vi "Inform.vi"(8 "error in (no error)":errorcluster, 10 "Message in":refnum<class "InformMessage.lvclass">, 11 "ServiceManager in":refnum<class "ServiceManager.lvclass">) -> (0 "error out":errorcluster, 3 "ServiceManager out":refnum<class "ServiceManager.lvclass">)   [LabVIEW 2012, in "ServiceManager.lvclass"]
doc: "The inform method processes the command inform'. \n\nThe command inform' is used for obtaining the latest instance data of the class. It also handles the current state of the observee and sets the 'ready' flag for the observee."
uses:
  ServiceManager.lvclass
  Murmex/LabVIEW/Murmex/InformMessage/InformMessage.lvclass
  Murmex/LabVIEW/Murmex/Murmex/Murmex.lvclass
  Murmex/LabVIEW/Murmex/Murmex/status_enum.ctl
  ServiceManager.lvclass/ServiceManager.ctl
  boot_parameters_cluster.ctl
  Murmex/LabVIEW/Murmex/Murmex/component_specification_cluster.ctl
  Murmex/LabVIEW/Murmex/GenericMessage/GenericMessage.lvclass
  Murmex/LabVIEW/Murmex/Message/Message.lvclass
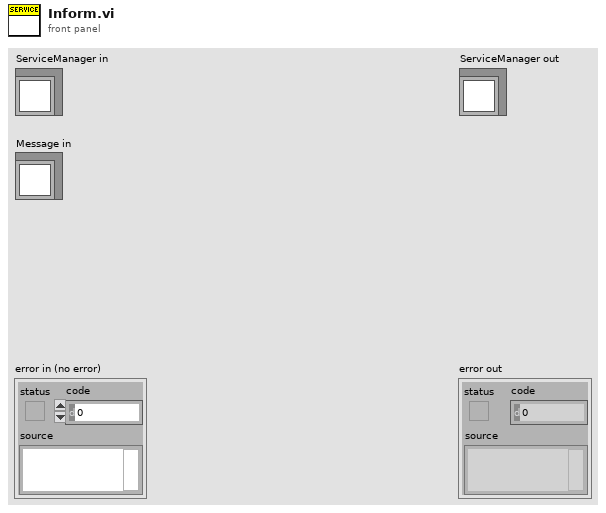
[diagram p1: front panel]
types:
  T1 = typedef "Murmex.lvlib/Murmex.lvclass/status_enum.ctl" = enum16{"ready", "warning", "error", "shutting down", "initialising"}
  T2 = typedef "ServiceManager.lvclass/boot_parameters_cluster.ctl" = cluster{"component specification":T3, "search paths":cluster{"path":string[]}}
  T3 = typedef "Murmex.lvlib/Murmex.lvclass/component_specification_cluster.ctl" = cluster{"name":string, "language":string, "host name":string, "id":string}
  T4 = typedef "ServiceManager.lvclass/loaded_components_cluster.ctl" = cluster{"component specification":T3, "booted?":bool, "status":T1, "last seen?":timestamp}
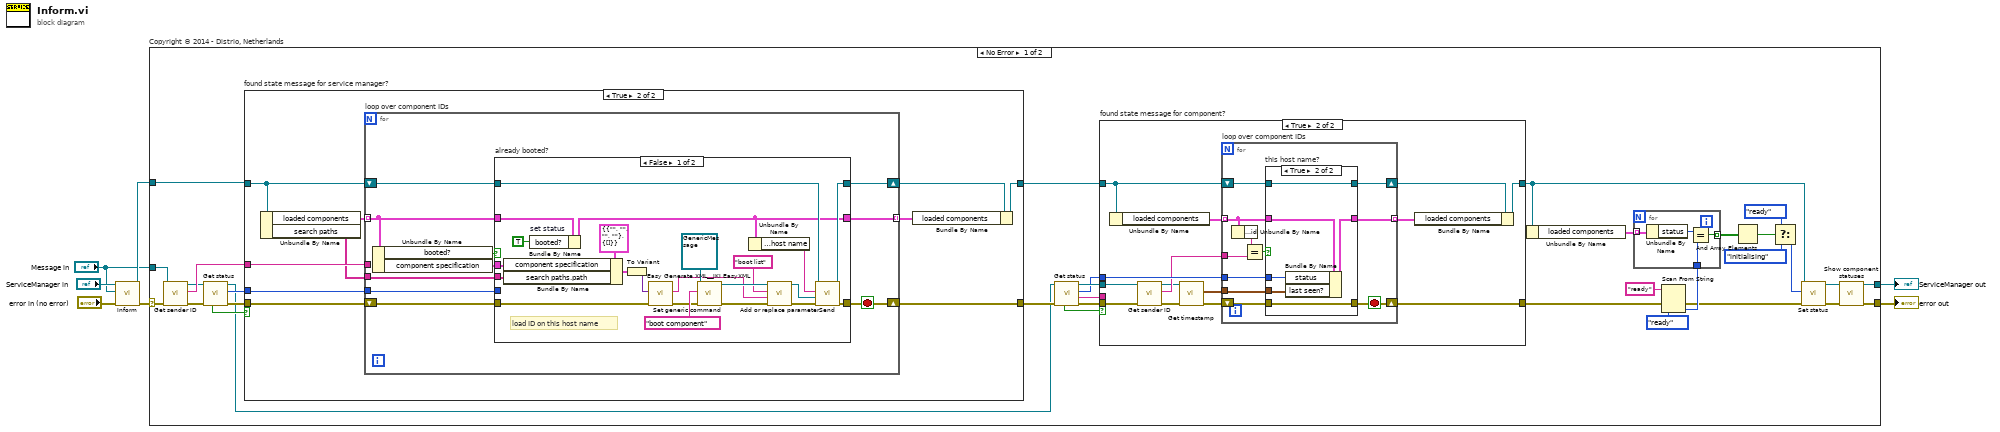
[diagram p0: block diagram]
diagram:
  n1 = call-parent "Inform.vi"("error in (no error)"="error in (no error)", "Message in"="Message in", "Murmex in"="ServiceManager in") -> ("error out"=w3:errorcluster, "Murmex out"=w2:refnum<class "ServiceManager.lvclass">)  [unwired: 7 in]
  n2 = case "Copyright © 2014 - Distrio, Netherlands" shown="No Error" w3 {
    selector: w3 -> [w39 w129]
    tunnel: [w23 w129] -> w5
    tunnel: [w24 w128] -> w4
    tunnel: "Message in" -> [w12 _]
    tunnel: w2 -> [w38 w128]
    frame No Error {
      n3 = call "Get sender ID.vi"("error in (no error)"=w39, "Message in"=w12) -> ("error out"=w21:errorcluster, "sender"=w40:string, "Message out"=w22:refnum<class "InformMessage.lvclass">)  [unwired: 7 in]
      n4 = call "Get status.vi"("error in (no error)"=w21, "Message in"=w22) -> ("error out"=w20:errorcluster, "status"=w19:T1, "Message out"=w10:refnum<class "InformMessage.lvclass">, "found?"=w18:bool)  [unwired: 4 in, 2 out]
      n5 = case "found state message for service manager?" shown="True" w18 {
        tunnel: w19 -> [_ w90]
        tunnel: [w82 w84] -> w16
        tunnel: w20 -> [w82 w85]
        tunnel: w40 -> [_ w92]
        tunnel: [w81 w88] -> w31
        tunnel: w38 -> [w81 w86]
        frame False {
        }
        frame True {
          n6 = Unbundle By Name(w86) -> ("loaded components"=w91:T4[], "search paths"=w83:string[])
          n7 = for "loop over component IDs" {
            tunnel: w91 -> [w101] mode=indexing
            tunnel: w92 -> [_]
            tunnel: w90 -> [w102]
            tunnel: [w100] -> w89 mode=indexing
            shift-right: [w98] -> w87
            shift-left: w86 -> [w99]
            shift-right: [w95] -> w84
            shift-left: w85 -> [w96]
            tunnel: w83 -> [w97]
            stop <- w95 stop-if-true
            n8 = Unbundle By Name(w101) -> ("booted?"=w94:bool, "component specification"=w93:T3)
            n9 = case "already booted?" shown="False" w94 {
              tunnel: w102 -> [_ _]
              tunnel: w101 -> [w124 w127]
              tunnel: w97 -> [w122 _]
              tunnel: w96 -> [w119 w125]
              tunnel: w99 -> [w118 w126]
              tunnel: [w117 w126] -> w98
              tunnel: [w116 w125] -> w95
              tunnel: [w115 w127] -> w100
              tunnel: w93 -> [w113 _]
              frame False {
                # "load ID on this host name"
                n10 = Bundle By Name(cluster=T2 {"component specification"={"name"="", "language"="", "host name"="", "id"=""}, "search paths"={"path"=[]}} ("boot parameters"), "component specification"=w113, "search paths.path"=w122) -> (w120:T2)
                n11 = Bundle By Name "set status"(cluster=w124, "booted?"=TRUE) -> (w115:T4)
                n12 = To Variant(anything=w120) -> (Variant=w121:variant)
                n13 = call <vilib>:"Easy Generate XML__JKI EasyXML.vi"("error in (no error)"=w119, "LabVIEW Data"=w121) -> ("error out"=w110:errorcluster, "XML String"=w104:string)  [unwired: 8 in]
                n14 = call "Set generic command.vi"("error in (no error)"=w110, "generic command"="boot component" ("command string"), "GenericMessage in"=refnum<class "GenericMessage.lvclass"> refnum ("GenericMessage.lvclass")) -> ("error out"=w107:errorcluster, "GenericMessage out"=w109:refnum<class "GenericMessage.lvclass">)  [unwired: 7 in]
                n15 = Unbundle By Name(w115) -> ("component specification.host name"=w114:string)
                n16 = call "Add or replace parameter.vi"("error in (no error)"=w107, "value"=w104, "name"="boot list", "Message in"=w109) -> ("error out"=w106:errorcluster, "Message out"=w108:refnum<class "GenericMessage.lvclass">)  [unwired: 6 in]
                n17 = call "Send.vi"("error in (no error)"=w106, "Message"=w108, "recipient"=w114, "Murmex in"=w118) -> ("error out"=w116:errorcluster, "Murmex out"=w117:refnum<class "ServiceManager.lvclass">)  [unwired: 6 in]
              }
              frame True {
                # "don't boot twice"
              }
            }
          }
          n18 = Bundle By Name(cluster=w87, "loaded components"=w89) -> (w88:refnum<class "ServiceManager.lvclass">)
        }
      }
      n19 = call "Get status.vi"("error in (no error)"=w16, "Message in"=w10) -> ("error out"=w15:errorcluster, "details"=w11:string, "status"=w13:T1, "Message out"=w14:refnum<class "InformMessage.lvclass">, "found?"=w17:bool)  [unwired: 4 in, 1 out]
      n20 = case "found state message for component?" shown="True" w17 {
        tunnel: w13 -> [_ w55]
        tunnel: [w42 w50] -> w9
        tunnel: w15 -> [w42 w44]
        tunnel: [w41 w53] -> w8
        tunnel: w31 -> [w41 w51]
        tunnel: w14 -> [_ w46]
        tunnel: w11 -> [_ _]
        frame False {
        }
        frame True {
          n21 = Unbundle By Name(w51) -> ("loaded components"=w56:T4[])
          n22 = call "Get sender ID.vi"("error in (no error)"=w44, "Message in"=w46) -> ("error out"=w43:errorcluster, "sender"=w47:string, "Message out"=w45:refnum<class "InformMessage.lvclass">)  [unwired: 7 in]
          n23 = call "Get timestamp.vi"("error in (no error)"=w43, "Message in"=w45) -> ("error out"=w49:errorcluster, "timestamp"=w48:timestamp)  [unwired: 7 in, 1 out]
          n24 = for "loop over component IDs" {
            tunnel: w56 -> [w63] mode=indexing
            tunnel: w47 -> [w67]
            tunnel: w55 -> [w64]
            tunnel: [w62] -> w54 mode=indexing
            shift-right: [w60] -> w52
            shift-left: w51 -> [w61]
            shift-right: [w58] -> w50
            shift-left: w49 -> [w59]
            tunnel: w48 -> [w57]
            stop <- w58 stop-if-true
            n25 = Unbundle By Name(w63) -> ("component specification.id"=w65:string)
            n26 = Equal?(x=w65, y=w67) -> (x = y?=w66:bool)
            n27 = case "this host name?" shown="True" w66 {
              tunnel: w64 -> [_ w71]
              tunnel: w63 -> [w70 w76]
              tunnel: [w70 w74] -> w62
              tunnel: w61 -> [w69 w75]
              tunnel: [w69 w75] -> w60
              tunnel: w59 -> [w68 w72]
              tunnel: [w68 w72] -> w58
              tunnel: w57 -> [_ w73]
              frame False {
              }
              frame True {
                n28 = Bundle By Name ("set boot\nstatus")(cluster=w76, "status"=w71, "last seen?"=w73) -> (w74:T4)
              }
            }
          }
          n29 = Bundle By Name(cluster=w52, "loaded components"=w54) -> (w53:refnum<class "ServiceManager.lvclass">)
        }
      }
      n30 = Unbundle By Name(w8) -> ("loaded components"=w37:T4[])
      n31 = Scan From String(input string="ready", error in=w9, default 1=status_enum."ready" ("y")) -> (error out=w27:errorcluster, output 1=w28:T1)  [unwired: 2 in, 2 out]
      n32 = for {
        tunnel: w37 -> [w80] mode=indexing
        tunnel: [w77] -> w36 mode=indexing
        tunnel: w28 -> [w79]
        n33 = Unbundle By Name(w80) -> ("status"=w78:T1)
        n34 = Equal?(x=w78, y=w79) -> (x = y?=w77:bool)
      }
      n35 = And Array Elements(Boolean array=w36) -> (logical AND=w34:bool)
      n36 = Select(t=status_enum."ready" ("status"), s=w34, f=status_enum."initialising" ("status")) -> (s? t:f=w32:T1)
      n37 = call "Set status.vi"("error in (no error)"=w27, "status"=w32, "Murmex in"=w8) -> ("error out"=w26:errorcluster, "Murmex out"=w25:refnum<class "ServiceManager.lvclass">)  [unwired: 7 in]
      n38 = call-dynamic "Show component statuses.vi"("error in (no error)"=w26, "ServiceManager in"=w25) -> ("error out"=w23:errorcluster, "ServiceManager out"=w24:refnum<class "ServiceManager.lvclass">)  [unwired: 8 in]
    }
    frame Error {
    }
  }
  "error out" <- w5
  "ServiceManager out" <- w4
